vi "Call Palette View.vi"(9 "Theme Mode":u16(ring) items=["Light Theme", "Light Medium Contrast", "Light High Contrast", "Dark Theme", "Dark Medium Contrast", "Dark High Constrast"], 10 "VI ref in":refnum<vi>, 11 "Material Theme":refnum<class "Material Theme.lvclass">) -> (0 "error out":errorcluster, 2 "VI ref":refnum<vi>)   [LabVIEW 2021]
doc: "Call and Forget the VIEW-Palette VI so that it can run in parallel for user interaction.\n\n<b>Code Developed By:</b> +\nDaniel Coons +\nTechnology Service Corporation +\nwww.tsc.com/atcs"
uses:
  Material-Scheme/Material-Scheme.lvclass
  Material Theme/Material Theme.lvclass
  Material-Scheme/View-User Colors.vi
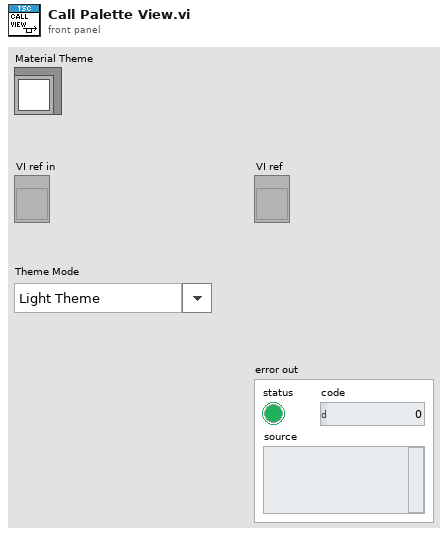
[diagram p1: front panel]
types:
  T1 = enum32{"Invalid", "Standard", "Closed", "Hidden", "Minimized", "Maximized"}
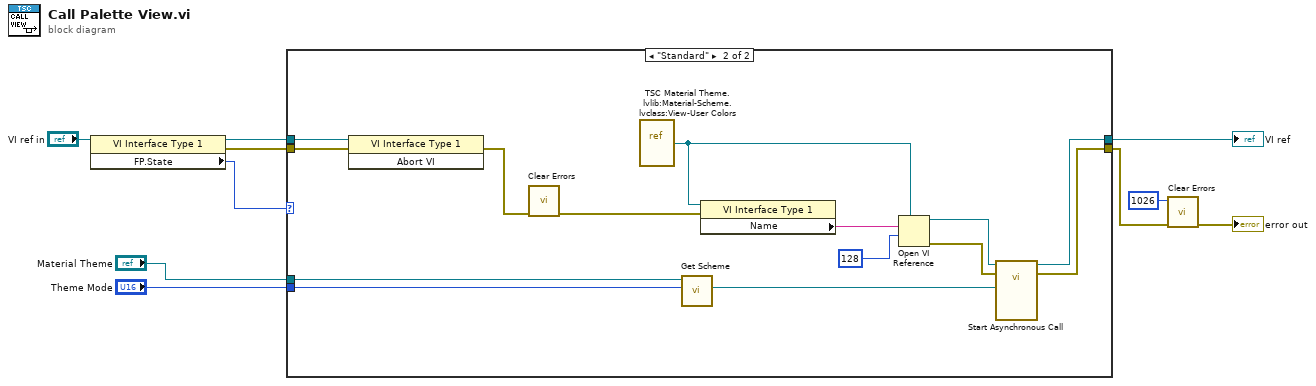
[diagram p0: block diagram]
diagram:
  n1 = property class="VI Interface Type 1"(reference="VI ref in") -> (reference out=w3:refnum<vi>, error out=w9:errorcluster, "FP.State"=w2:T1)  [unwired: 1 in]
  n2 = case shown="\"Standard\"" w2 {
    tunnel: "Material Theme" -> [_ w21]
    tunnel: "Theme Mode" -> [_ w20]
    tunnel: w3 -> [w11 w19]
    tunnel: [w11 w13] -> w4
    tunnel: [w12 w25] -> w10
    tunnel: w9 -> [w12 w22]
    frame Default {
    }
    frame "Standard" {
      n3 = invoke class="VI Interface Type 1" method="Abort VI"(reference=w19, error in=w22) -> (error out=w24:errorcluster)  [unwired: 1 in, 2 out]
      n4 = call <vilib>:"Clear Errors.vi"("error in (no error)"=w24) -> ("error out"=w23:errorcluster)  [unwired: 5 in, 1 out]
      n5 = vi-ref "TSC Material Theme.lvlib:Material-Scheme.lvclass:View-User Colors.vi"() -> (w14:refnum<vi>)
      n6 = call "Get Scheme.vi"("Theme"=w20, "Material Theme in"=w21) -> ("Material-Scheme"=w18:refnum<class "Material-Scheme.lvclass">)  [unwired: 7 in, 2 out]
      n7 = property class="VI Interface Type 1"(reference=w14, error in=w23) -> ("Name"=w17:string)  [unwired: 2 out]
      n8 = Open VI Reference(type specifier VI Refnum (for type only)=w14, vi path=w17, options=128) -> (vi reference=w15:refnum<vi>, error out=w26:errorcluster)  [unwired: 3 in]
      n9 = call-by-ref "Start Asynchronous Call"(reference=w15, error in=w26, "Material-Scheme.lvclass"=w18) -> (reference out=w13:refnum<vi>, error out=w25:errorcluster)  [unwired: 11 in]
    }
  }
  "VI ref" <- w4
  n10 = call <vilib>:"Clear Errors.vi"("error in (no error)"=w10, "specific error code to clear (0: all)"=1026) -> ("error out"=→"error out":errorcluster)  [unwired: 4 in, 1 out]
